vi "Destroy Event References.vi"(8 "error in":errorcluster, 11 "Event References":T1) -> (0 "error out":errorcluster)   [LabVIEW 2024, in "serenial.io-ase.lvlib" / "ase.lvclass"]
doc: "<B>Destroy the Event References.</B>\n\nThis VI will still operate when there is an error at the error-in terminal."
uses:
  ase.lvclass
  Event References.ctl
  Standard Output.ctl
  Standard Error.ctl
  Did Exit.ctl
  ase.lvclass/ase.ctl
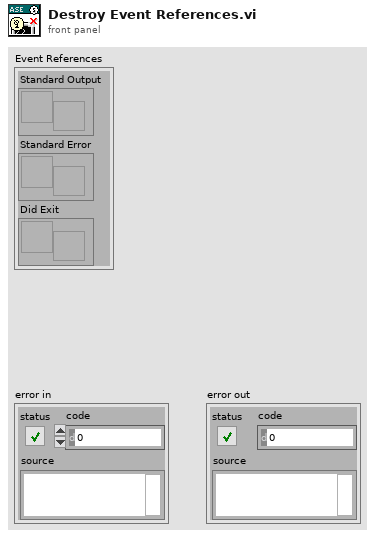
[diagram p1: front panel]
types:
  T1 = typedef "serenial.io-ase.lvlib/ase.lvclass/Event References.ctl" = cluster{"Standard Output":refnum<user-event>, "Standard Error":refnum<user-event>, "Did Exit":refnum<user-event>}
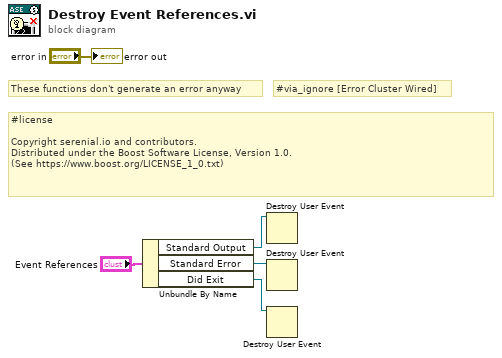
[diagram p0: block diagram]
diagram:
  # "#license\n\nCopyright serenial.io and contributors.\nDistributed under the Boost Software License, Version 1.0.\n(See https://www.boost.org/LICENSE_1_0.txt)"
  # "#via_ignore [Error Cluster Wired]"
  # "These functions don't generate an error anyway"
  n1 = Unbundle By Name("Event References") -> ("Standard Output"=w5:refnum<user-event>, "Standard Error"=w4:refnum<user-event>, "Did Exit"=w3:refnum<user-event>)
  n2 = Destroy User Event(user event=w5) -> ()  [unwired: 1 in, 1 out]
  n3 = Destroy User Event(user event=w4) -> ()  [unwired: 1 in, 1 out]
  n4 = Destroy User Event(user event=w3) -> ()  [unwired: 1 in, 1 out]
  "error out" <- "error in"
